vi "XIPIN_3GPP_Turbo_Encoder_5_0.vi"   [LabVIEW 2017]
doc: "The Turbo encoder LogiCORE from Xilinx is a high-speed, compact Turbo Encoder which meets the 3GPP specification. The core is delivered through the Xilinx CORE Generator System and integrates seamlessly with the Xilinx design flow.\n------------------------------------\n<b>Need License</b> : Yes"
uses:
  <vilib>/rvi/XilinxIP/XIPIN_XNode/niFpgaXIPIN.xnode
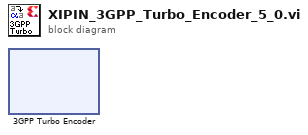
[diagram p0: block diagram]
diagram:
  n1 = xnode ("3GPP Turbo Encoder")() -> ()
